vi "Serialize U32.vi"(3 "data":u32) -> (1 "bytes":u8[](array[numeric]))   [LabVIEW 2020, in "NI_SFTP.lvlib" / "Low Level Connection.lvclass"]
uses:
  <vilib>/net/SFTP/Low Level Connection/Low Level Connection.lvclass
  <vilib>/Bit Manipulation/wrappers/Words To Network-Order Bytes/Words To Network-Order Bytes U32.vi
  <vilib>/Bit Manipulation/NI_Bit Manipulation.lvlib
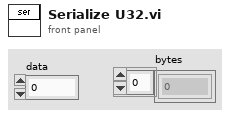
[diagram p1: front panel]
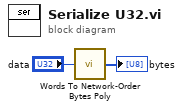
[diagram p0: block diagram]
diagram:
  n1 = call-poly <vilib>:"Words To Network-Order Bytes Poly.vi"("word"="data") -> ("bytes"=→"bytes":u8[])
